vi "CombineData.vi"(4 "FPGAData":dbl[](array[numeric]), 6 "PXI6733Output":dbl[](array[numeric]), 9 "PXI6254Data":dbl[](array[numeric]), 10 "PXI6123Data":dbl[](array[numeric]), 11 "PXI6122Data":dbl[](array[numeric])) -> (3 "Array":dbl[](array[numeric]))   [LabVIEW 2011]
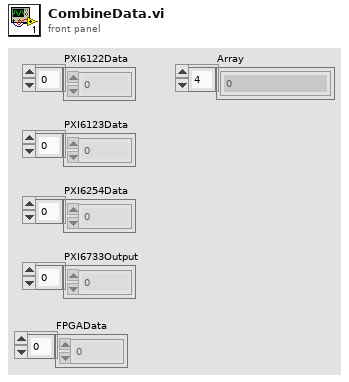
[diagram p1: front panel]
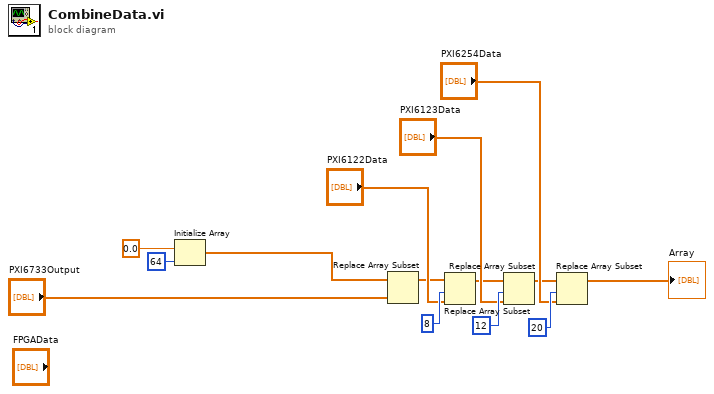
[diagram p0: block diagram]
diagram:
  n1 = Initialize Array(0.0, 64 ("dimension size")) -> (w1:dbl[])
  n2 = Replace Array Subset(array=w1, new element="PXI6733Output") -> (w4:dbl[])  [unwired: 1 in]
  n3 = Replace Array Subset(array=w4, new element="PXI6122Data", index=8) -> (w7:dbl[])
  n4 = Replace Array Subset(array=w7, new element="PXI6123Data", index=12) -> (w10:dbl[])
  n5 = Replace Array Subset(array=w10, new element="PXI6254Data", index=20) -> (→"Array":dbl[])
